vi "PID Motors.vi"(4 "input B":dbl, 5 "Speed B":dbl(slide)=-0.016713091922005565 scale=-2.0..2.0, 6 "input A":dbl, 7 "Speed A":dbl(slide)=-0.016713091922005565 scale=-2.0..2.0) -> (0 "output B":dbl, 1 "PID B":cluster{"Setpoint":dbl, "dx/dt":dbl}(graph), 2 "output A":dbl, 3 "PID A":cluster{"Setpoint":dbl, "dx/dt":dbl}(graph))   [LabVIEW 2017]
panel:
  in  "PID gains":T1={"proportional gain (Kc)"=0.015, "integral time (Ti, min)"=0.003, "derivative time (Td, min)"=0.0} {"derivative time (Td, min)" format="%.6f"; "integral time (Ti, min)" format="%.6f"; "proportional gain (Kc)" format="%.6f"}
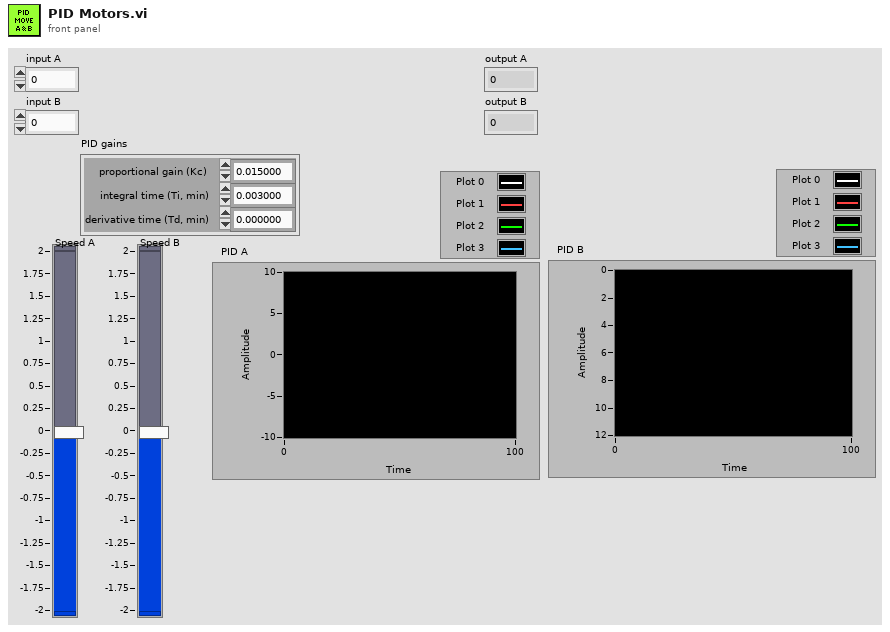
[diagram p1: front panel]
types:
  T1 = cluster{"proportional gain (Kc)":dbl, "integral time (Ti, min)":dbl, "derivative time (Td, min)":dbl}
  T2 = cluster{"Setpoint":dbl, "output":dbl, "dx/dt":dbl}
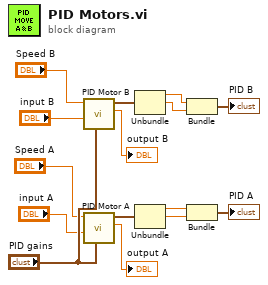
[diagram p0: block diagram]
diagram:
  n1 = call "PID Motor B.vi"("PID gains"="PID gains", "input"="input B", "Setpoint B0"="Speed B") -> ("output"=→"output B":dbl, "Speed B0"=w14:T2)  [unwired: 3 in, 4 out]
  n2 = call "PID Motor A.vi"("PID gains"="PID gains", "input"="input A", "Setpoint A0"="Speed A") -> ("output"=→"output A":dbl, "Speed A0"=w13:T2)  [unwired: 3 in, 4 out]
  n3 = Unbundle(w14) -> ("Setpoint"=w11:dbl, "output"=w1:dbl)  [unwired: 1 out]
  n4 = Unbundle(w13) -> ("Setpoint"=w12:dbl, "output"=w2:dbl)  [unwired: 1 out]
  n5 = Bundle("Setpoint"=w11, "output"=w1) -> (→"PID B":cluster{"Setpoint":dbl, "output":dbl})  [unwired: 1 in]
  n6 = Bundle("Setpoint"=w12, "output"=w2) -> (→"PID A":cluster{"Setpoint":dbl, "output":dbl})  [unwired: 1 in]
